vi "wielo_wątki.vi"() -> ()   [LabVIEW 2018]
uses:
  <vilib>/sound2/lvsound2.llb/Sound Data Format.ctl
  lab6/stany.ctl
  <vilib>/sound2/lvsound2.llb/Sampling Mode.ctl
  <vilib>/sound2/lvsound2.llb/Sound Input Read (DBL).vi
panel:
  out "Waveform Graph":waveform(dbl)[](graph)
  in  "STOP":bool
  in  "sound format":T1={"sample rate (S/s)"=22050.0, "number of channels"=2, "bits per sample"=16}
  in  "num of sampl":i32
  in  "Play":bool
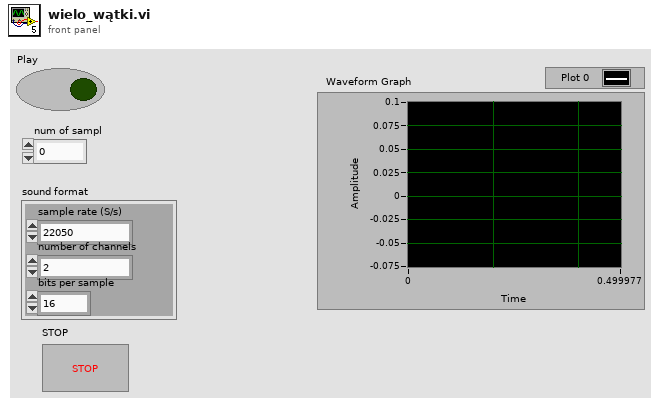
[diagram p1: front panel]
types:
  T1 = typedef "Sound Data Format.ctl" = cluster{"sample rate (S/s)":dbl, "number of channels":i32, "bits per sample":i32}
  T2 = typedef "stany.ctl" = enum16{"Idle", "Initialization", "Acquisition", "End"}
  T3 = cluster{"Play":bool, "num of sampl":i32, "sound format 2":T1}
  T4 = cluster{"Play":bool, "num of sampl":i32, "sound format":T1}
  T5 = typedef "Sampling Mode.ctl" = i32
  T6 = typedef "Sound Input Task ID.ctl" = u32
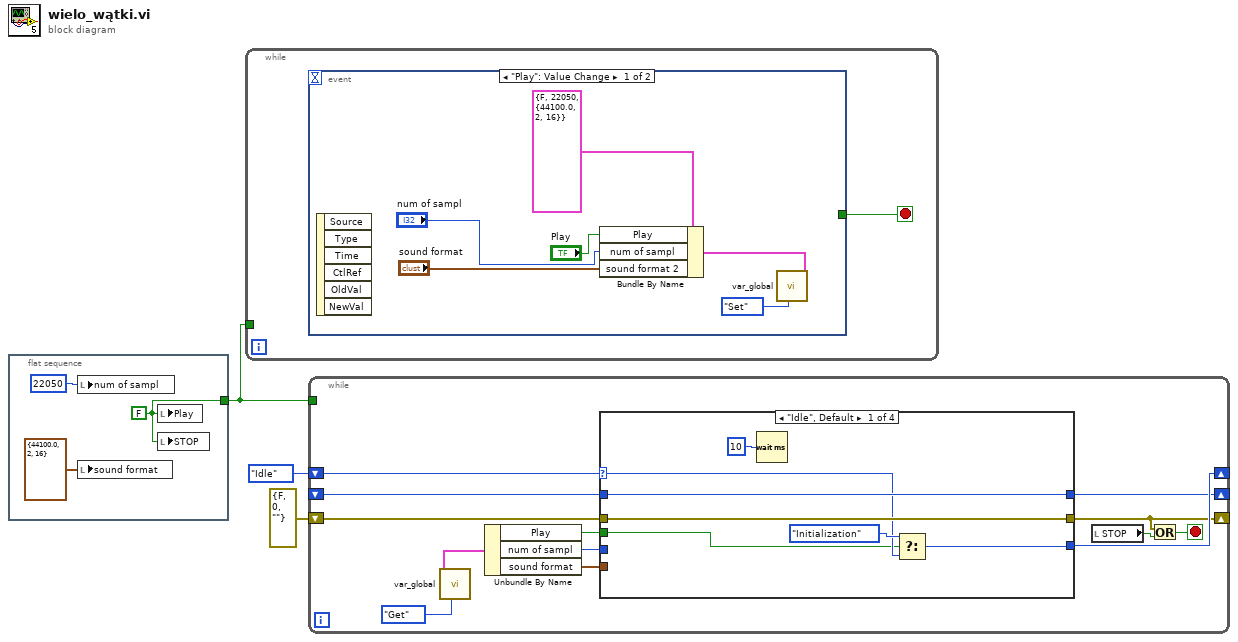
[diagram p0: block diagram]
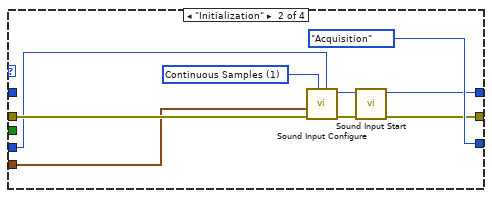
[diagram p2: hidden frame]
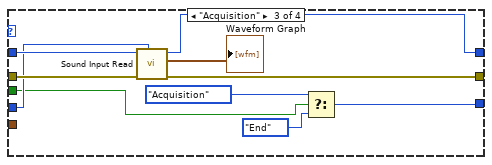
[diagram p3: hidden frame]
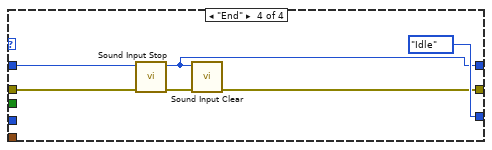
[diagram p4: hidden frame]
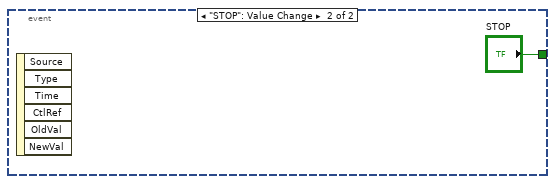
[diagram p5: hidden frame]
diagram:
  n1 = flat-sequence {
    tunnel: [w4] -> w1
    frame #0 {
      w4 = FALSE
      n2 = local write "num of sampl"(22050 ("num of sampl")) -> ()
      n3 = local write "sound format"(T1 {"sample rate (S/s)"=44100.0, "number of channels"=2, "bits per sample"=16} ("sound format 2")) -> ()
      n4 = local write "Play"(w4) -> ()
      n5 = local write "STOP"(w4) -> ()
    }
  }
  n6 = while {
    tunnel: w1 -> [_]
    stop <- w7 stop-if-true
    n7 = event shown="[0] \"Play\": Value Change" {
      selector: _ -> [_ _]
      dyn-events: _ -> [_ _]
      timeout: _ -> [_ _]
      tunnel: [_ "STOP"] -> w7
      event "Play": Value Change {
        n8 = event-data() -> ()  [unwired: 1 in, 6 out]
        n9 = Bundle By Name(cluster=T3 {"Play"=FALSE, "num of sampl"=22050, "sound format 2"={"sample rate (S/s)"=44100.0, "number of channels"=2, "bits per sample"=16}} ("input cluster"), "Play"="Play", "num of sampl"="num of sampl", "sound format 2"="sound format") -> (w11:T3)
        n10 = call "var_global.vi"("Param in"=w11, "Action"=enum16{"Set", "Get"}."Set") -> ()  [unwired: 9 in, 1 out]
      }
      event "STOP": Value Change {
        n11 = event-data() -> ()  [unwired: 1 in, 6 out]
      }
    }
  }
  n12 = while {
    shift-right: [w26] -> _
    shift-left: stany."Idle" ("Enum") -> [w27]
    shift-right: [w22] -> _
    shift-left: errorcluster {"status"=FALSE, "code"=0, "source"=""} ("error out") -> [w23]
    shift-right: [w25] -> _
    shift-left: _ -> [w24]
    tunnel: w1 -> [_]
    stop <- w16 stop-if-true
    n13 = call "var_global.vi"("Action"=enum16{"Set", "Get"}."Get") -> ("Param out"=w20:T4)  [unwired: 10 in]
    n14 = Unbundle By Name(w20) -> ("Play"=w19:bool, "num of sampl"=w17:i32, "sound format"=w18:T1)
    n15 = case shown="\"Idle\", Default" w27 {
      selector: w27 -> [w30 _ _ _]
      tunnel: [w33 stany."Acquisition" w51 stany."Idle"] -> w26
      tunnel: [w32 w40 w48 w55] -> w25
      tunnel: w23 -> [w31 w38 w49 w57]
      tunnel: w24 -> [w32 _ w50 w56]
      tunnel: [w31 w37 w47 w54] -> w22
      tunnel: w19 -> [w28 _ w45 _]
      tunnel: w17 -> [_ w35 w46 _]
      tunnel: w18 -> [_ w36 _ _]
      frame "Idle", Default {
        n16 = Wait (ms)(milliseconds to wait=u32 10) -> ()  [unwired: 1 out]
        n17 = Select(t=stany."Initialization", s=w28, f=w30) -> (s? t:f=w33:T2)
      }
      frame "Initialization" {
        w39 = T5 1 items=["Finite Samples", "Continuous Samples"] ("sample mode")
        n18 = call <vilib>:"Sound Input Configure.vi"("number of samples/ch"=w35, "sample mode"=w39, "error in (no error)"=w38, "sound format"=w36) -> ("error out"=w42:errorcluster, "task ID"=w43:T6)  [unwired: 6 in]
        n19 = call <vilib>:"Sound Input Start.vi"("error in (no error)"=w42, "task ID"=w43) -> ("error out"=w37:errorcluster, "task ID out"=w40:T6)  [unwired: 8 in]
      }
      frame "Acquisition" {
        n20 = call-poly <vilib>:"Sound Input Read.vi"("number of samples/ch"=w46, "error in (no error)"=w49, "task ID"=w50) -> ("error out"=w47:errorcluster, "data"=→"Waveform Graph":waveform(dbl)[], "task ID out"=w48:T6)  [unwired: 6 in]
        n21 = Select(t=stany."Acquisition", s=w45, f=stany."End") -> (s? t:f=w51:T2)
      }
      frame "End" {
        n22 = call <vilib>:"Sound Input Stop.vi"("error in (no error)"=w57, "task ID"=w56) -> ("error out"=w59:errorcluster, "task ID out"=w55:T6)  [unwired: 8 in]
        n23 = call <vilib>:"Sound Input Clear.vi"("error in (no error)"=w59, "task ID"=w55) -> ("error out"=w54:errorcluster)  [unwired: 9 in]
      }
    }
    n24 = local read "STOP"() -> (w15:bool)
    n25 = Or(x=w22, y=w15) -> (x .or. y?=w16:bool)
  }
